vi "New Mode Code.vi"(6 "direction (Tx)":i32(ring) items=["Tx", "Rx"], 7 "messageBufferIDRef (-1)":i32=-1, 8 "error in":errorcluster, 9 "modeCodeNumber":i8, 10 "ModeCode Config":T1 {"elapseMinOrMax" items=["Elapsetime", "Mintime", "Maxtime"]; "timeOrHitCount" items=["Time", "HitCount"]; "dataWipe" items=["Zeroes", "CWD", "Item123", "None"]}, 11 "name":string) -> (0 "error out":errorcluster, 3 "modeCode out":refnum<k24>)   [LabVIEW 2020, in "Ballard_1553_Hardware_ni.lvlib"]
uses:
  Ballard_1553_Hardware_ni.lvlib
  C:/Users/Administrator/Desktop/GIT/Ballard-MIL-STD-1553-Custom-Device/Source/System Explorer/SubVIs/Parse XML Ballard/1.2/BTIXML_SerDes.dll
  Ballard-MIL-STD-1553-Custom-Device/Source/System Explorer/SubVIs/Parse XML Ballard/1.2/BTIXML_SerDes.dll
  _typedefs/modeCode_type.ctl
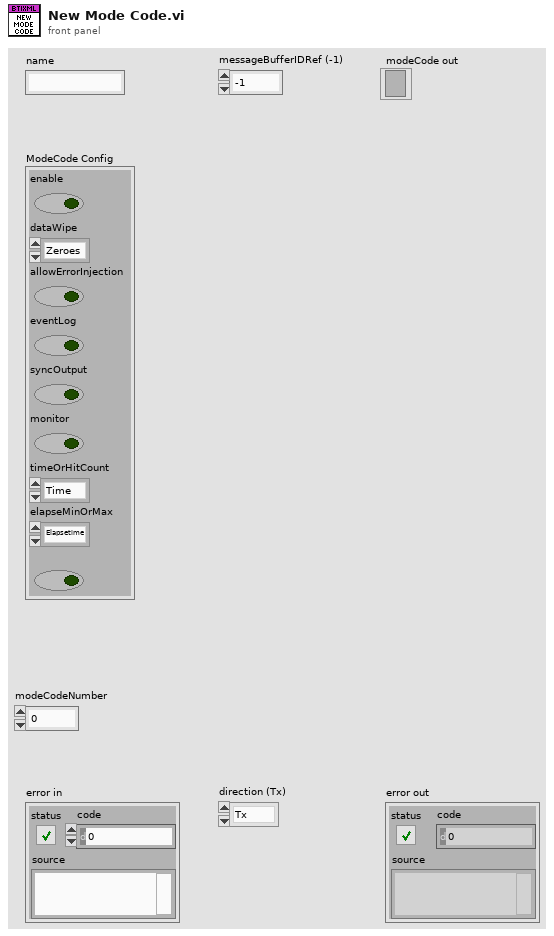
[diagram p1: front panel]
types:
  T1 = typedef "Ballard_1553_Hardware_ni.lvlib/modeCode_type.ctl" = cluster{"enable":bool, "dataWipe":i32, "allowErrorInjection":bool, "eventLog":bool, "syncOutput":bool, "monitor":bool, "timeOrHitCount":i32, "elapseMinOrMax":i32, "wrap":bool}
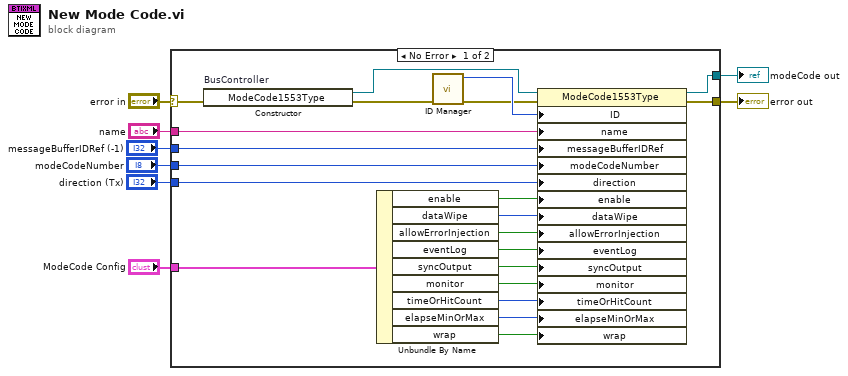
[diagram p0: block diagram]
diagram:
  n1 = case shown="No Error" "error in" {
    selector: "error in" -> [w29 w30]
    tunnel: [w28 w30] -> w7
    tunnel: [w27 _] -> w1
    tunnel: "ModeCode Config" -> [w22 _]
    tunnel: "name" -> [w21 _]
    tunnel: "direction (Tx)" -> [w20 _]
    tunnel: "modeCodeNumber" -> [w19 _]
    tunnel: "messageBufferIDRef (-1)" -> [w18 _]
    frame No Error {
      n2 = constructor on="BusController" class="ModeCode1553Type"(error in=w29) -> (reference out=w26:refnum<k24>, error out=w25:errorcluster)  [unwired: 2 in, 1 out]
      n3 = Unbundle By Name(w22) -> ("enable"=w17:bool, "dataWipe"=w16:i32, "allowErrorInjection"=w15:bool, "eventLog"=w14:bool, "syncOutput"=w13:bool, "monitor"=w12:bool, "timeOrHitCount"=w11:i32, "elapseMinOrMax"=w10:i32, "wrap"=w9:bool)
      n4 = call "ID Manager.vi"("error in"=w25) -> ("error out"=w23:errorcluster, "ID out"=w24:i32)  [unwired: 9 in]
      n5 = property class="ModeCode1553Type"(reference=w26, error in=w23, "ID"=w24, "name"=w21, "messageBufferIDRef"=w18, "modeCodeNumber"=w19, "direction"=w20, "enable"=w17, "dataWipe"=w16, "allowErrorInjection"=w15, "eventLog"=w14, "syncOutput"=w13, "monitor"=w12, "timeOrHitCount"=w11, "elapseMinOrMax"=w10, "wrap"=w9) -> (reference out=w27:refnum<k24>, error out=w28:errorcluster)
    }
    frame Error {
    }
  }
  "error out" <- w7
  "modeCode out" <- w1
